vi "温度采集并插入数据库.vi"(6 "目标温度":string(combo), 7 "数据显示1":string[][](table), 8 "错误输入（无错误）":errorcluster, 9 "实测温度":string, 10 "通道号":i32, 11 "VISA引用句柄输入":refnum<visa-resource-name>) -> (0 "错误输出":errorcluster, 1 "温度值s":dbl[](array[numeric]), 2 "数据显示2":string[][](table), 3 "VISA引用句柄输出":refnum<visa-resource-name>)   [LabVIEW 2015]
uses:
  <vilib>/Analysis/NI_AALBase.lvlib
  <vilib>/Analysis/baseanly.llb/Mean (DBL).vi
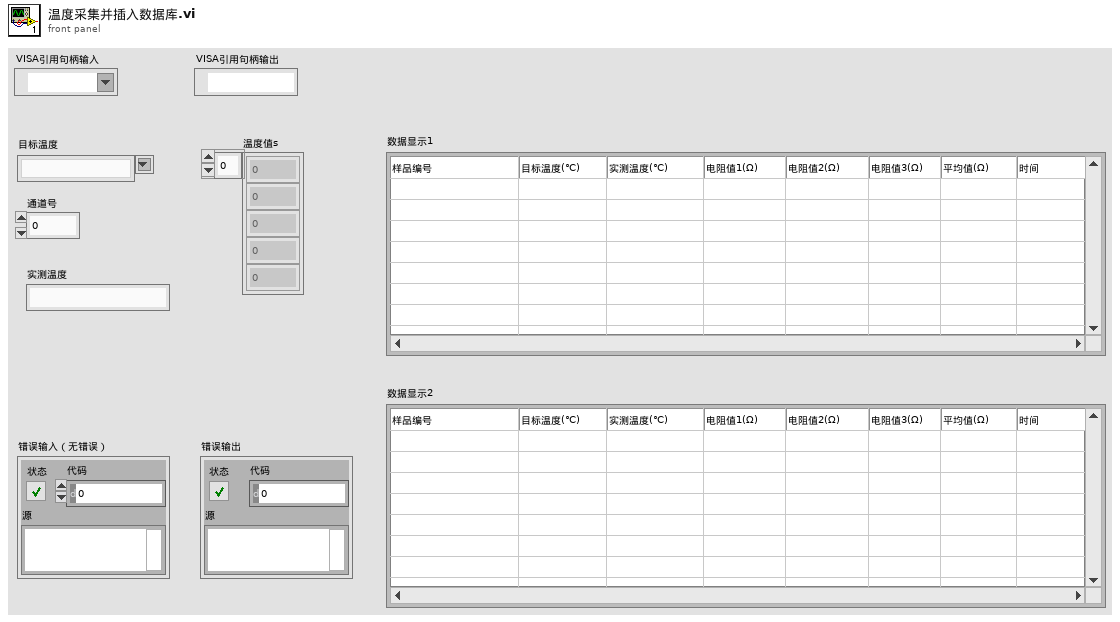
[diagram p1: front panel]
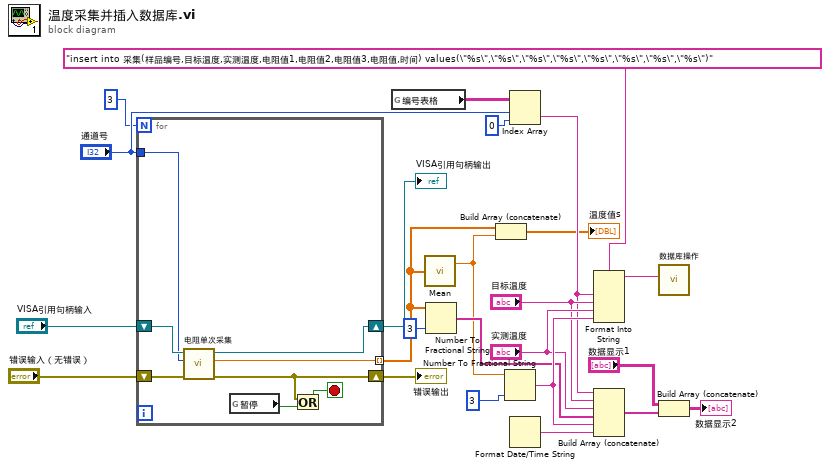
[diagram p0: block diagram]
diagram:
  n1 = for {
    N: 3 -> [_]
    shift-right: [w26] -> w19
    shift-left: "错误输入（无错误）" -> [w32]
    shift-right: [w30] -> w9
    shift-left: "VISA引用句柄输入" -> [w31]
    tunnel: "通道号" -> [w29]
    tunnel: [w28] -> w5 mode=indexing
    stop <- w25 stop-if-true
    n2 = call "电阻单次采集.vi"("错误输入（无错误）"=w32, "通道数"=w29, "VISA引用句柄输入"=w31) -> ("错误输出"=w26:errorcluster, "测量结果"=w28:dbl, "VISA引用句柄输出"=w30:refnum<visa-resource-name>)  [unwired: 5 in, 1 out]
    n3 = global read "全局.vi" "暂停"() -> (w27:bool)
    n4 = Or(x=w26, y=w27) -> (x .or. y?=w25:bool)
  }
  "错误输出" <- w19
  "VISA引用句柄输出" <- w9
  n5 = global read "全局.vi" "编号表格"() -> (w12:string[][])
  n6 = call-poly <vilib>:"Mean.vi"("X"=w5) -> ("mean"=w4:dbl)  [unwired: 1 out]
  n7 = Number To Fractional String(number=w5, precision (6)=i16 3 ("精度(6)")) -> (F-format string=w17:string[])  [unwired: 2 in]
  n8 = Build Array (concatenate)(w5, w4) -> (→"温度值s":dbl[])
  n9 = Number To Fractional String(number=w4, precision (6)=i16 3 ("精度(6)")) -> (F-format string=w22:string)  [unwired: 2 in]
  n10 = Index Array(array=w12, index (row)="通道号", index (col)=0 ("禁用的索引 (列)")) -> (element=w16:string)
  n11 = Format Date/Time String() -> (date/time string=w18:string)  [unwired: 3 in]
  n12 = Format Into String(format string="insert into 采集(样品编号,目标温度,实测温度,电阻值1,电阻值2,电阻值3,电阻值,时间) values(\"%s\",\"%s\",\"%s\",\"%s\",\"%s\",\"%s\",\"%s\",\"%s\")" ("SQL"), w16, "目标温度", "实测温度", w22) -> (resulting string=w15:string)  [unwired: 2 in, 1 out]
  n13 = Build Array (concatenate)(w16, "目标温度", "实测温度", w17, w22, w18) -> (w23:string[])
  n14 = call "数据库操作.vi"("SQL query"=w15) -> ()  [unwired: 9 in, 2 out]
  n15 = Build Array (concatenate)("数据显示1", w23) -> (→"数据显示2":string[][])
